vi "MB Serial Slave Communication.vi"(8 "error in (no error)":errorcluster, 9 "Timeout":u32=10000, 10 "Serial Parameters":T1 {"Slave Address" format="%.0x"}, 11 "VISA resource name":refnum<visa-resource-name>) -> (0 "error out":errorcluster, 3 "VISA resource name out":refnum<visa-resource-name>)   [LabVIEW 2011]
panel:
  # "VI Name: MB Serial Slave Communication.vi\nPurpose: MODBUS Slave Read.\nReentrant."
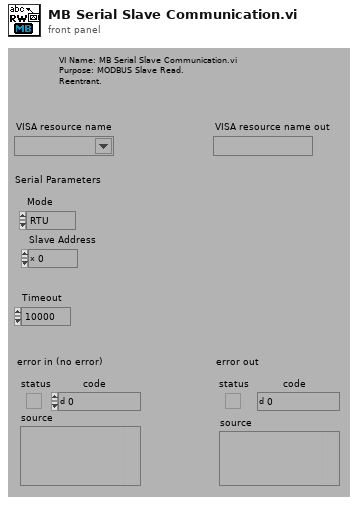
[diagram p1: front panel]
types:
  T1 = cluster{"Mode":enum16{"RTU", "ASCII"}, "Slave Address":u8}
  T2 = typedef "MB Modbus Data Unit.ctl" = cluster{"Function Code":u8, "Data":u8[]}
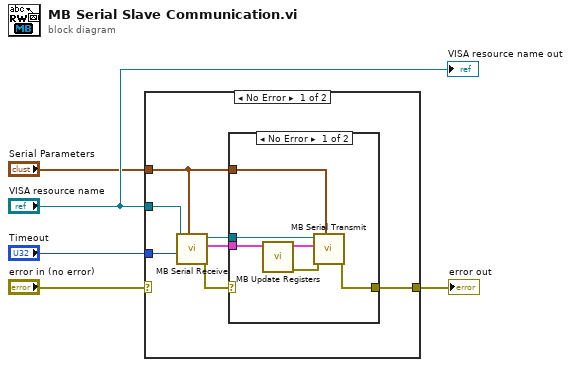
[diagram p0: block diagram]
diagram:
  n1 = case shown="No Error" "error in (no error)" {
    selector: "error in (no error)" -> [_ w20]
    tunnel: "VISA resource name" -> [w12 _]
    tunnel: [w11 w20] -> w5
    tunnel: "Timeout" -> [w9 _]
    tunnel: "Serial Parameters" -> [w6 _]
    frame No Error {
      n2 = call "MB Serial Receive.vi"("Serial Parameters"=w6, "Timeout"=w9, "VISA resource name"=w12) -> ("error out"=w7:errorcluster, "Modbus Data Unit"=w8:T2, "VISA resource name out"=w10:refnum<visa-resource-name>)  [unwired: 2 in, 4 out]
      n3 = case shown="No Error" w7 {
        selector: w7 -> [_ w19]
        tunnel: [w18 w19] -> w11
        tunnel: w10 -> [w17 _]
        tunnel: w6 -> [w15 _]
        tunnel: w8 -> [w14 _]
        frame No Error {
          n4 = call "MB Update Registers.vi"("Modbus Data Unit In"=w14) -> ("error out"=w16:errorcluster, "Modbus Data Unit Out"=w13:T2)  [unwired: 1 in, 8 out]
          n5 = call "MB Serial Transmit.vi"("Serial Parameters"=w15, "error in (no error)"=w16, "Modbus Data Unit"=w13, "VISA resource name"=w17) -> ("error out"=w18:errorcluster)  [unwired: 2 in, 5 out]
        }
        frame Error {
        }
      }
    }
    frame Error {
    }
  }
  "error out" <- w5
  "VISA resource name out" <- "VISA resource name"
